vi "Get Assertion Status From Test Case.vi"(11 "Test Case Test Double in":refnum<class "Test Case Test Double.lvclass">) -> (3 "Status":T1)   [LabVIEW 2020, in "LUnit Tests.lvlib" / "Assertion Result Test.lvclass"]
uses:
  Assertion Result Test.lvclass
  source/Framework/Result Classes/Assertion Result/Public/TypeDefs/Status.ctl
  Test Dummys/Test Case Test Double/Test Case Test Double.lvclass
  C:/Users/anton/Documents/GitHub/LUnit/source/Framework/Test Case/LUnit Test Case.lvclass
  source/Framework/Test Case/LUnit Test Case.lvclass/LUnit Test Case.ctl
  source/Framework/Result Classes/Test Case Result/Test Case Result.lvclass/Test Case Result.ctl
  source/Framework/Result Classes/Method Result/Method Result.lvclass/Method Result.ctl
  source/Framework/Test Case/LUnit Test Case.lvclass
  source/Framework/Result Classes/Test Case Result/Test Case Result.lvclass
  source/Framework/Result Classes/Method Result/Method Result.lvclass
  source/Framework/Result Classes/Assertion Result/Assertion Result.lvclass
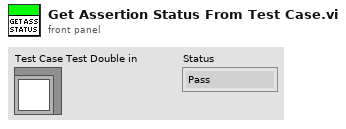
[diagram p1: front panel]
types:
  T1 = typedef "Assertion Result.lvclass/Status.ctl" = enum16{"Pass", "Fail", "Error", "Skipped", "Setup Error", "Broken", "Teardown Error"}
  T2 = map{string, refnum<class "Method Result.lvclass">}
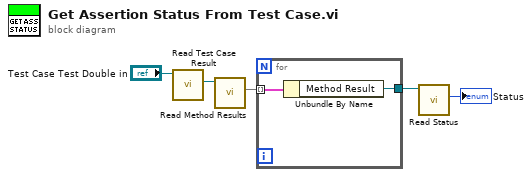
[diagram p0: block diagram]
diagram:
  n1 = call "Read Test Case Result.vi"("LUnit Test Case In"="Test Case Test Double in") -> ("Test Case Result"=w2:refnum<class "Test Case Result.lvclass">)  [unwired: 9 in, 1 out]
  n2 = call "Read Method Results.vi"("Test Case Result In"=w2) -> ("Method Results"=w3:T2)  [unwired: 9 in, 1 out]
  n3 = for {
    tunnel: [w7] -> w4
    tunnel: w3 -> [w6] mode=indexing
    n4 = Unbundle By Name(w6) -> ("Method Result"=w7:refnum<class "Method Result.lvclass">)
  }
  n5 = call "Read Status.vi"("Method Result In"=w4) -> ("Status"=→"Status":T1)  [unwired: 8 in, 2 out]
